vi "Unsigned_InRange_Coerce.vi"(9 "Min":dbl, 10 "Value":dbl, 11 "Max":dbl) -> (1 "In Range":bool, 3 "Clamped":dbl)   [LabVIEW 2013]
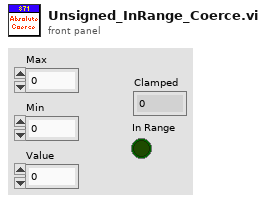
[diagram p1: front panel]
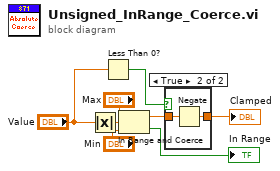
[diagram p0: block diagram]
diagram:
  n1 = Absolute Value(x="Value") -> (abs(x)=w8:dbl)
  n2 = Less Than 0?(x="Value") -> (x < 0?=w7:bool)
  n3 = In Range and Coerce(upper limit="Max", x=w8, lower limit="Min") -> (coerced(x)=w6:dbl, In Range?=→"In Range":bool)
  n4 = case shown="True" w7 {
    tunnel: w6 -> [w9 w11]
    tunnel: [w9 w10] -> w2
    frame False {
    }
    frame True {
      n5 = Negate(x=w11) -> (-x=w10:dbl)
    }
  }
  "Clamped" <- w2
